vi "Evaluate.vi"(0 "object in":refnum<class "BallInterception.lvclass">, 2 "Point":dbl[](array[numeric]), 3 "Ally?":bool, 4 "GameRef":refnum<data-value>, 5 "error in (no error)":errorcluster) -> (14 "object out":refnum<class "BallInterception.lvclass">, 16 "Evaluation":dbl, 19 "error out":errorcluster)   [LabVIEW 2023, in "BallInterception.lvclass"]
uses:
  BallInterception.lvclass
  Game_class/Game.lvclass
  BallInterception.lvclass/BallInterception.ctl
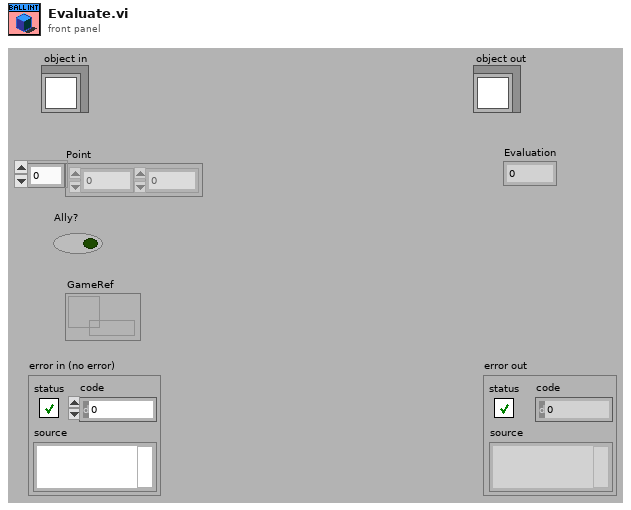
[diagram p1: front panel]
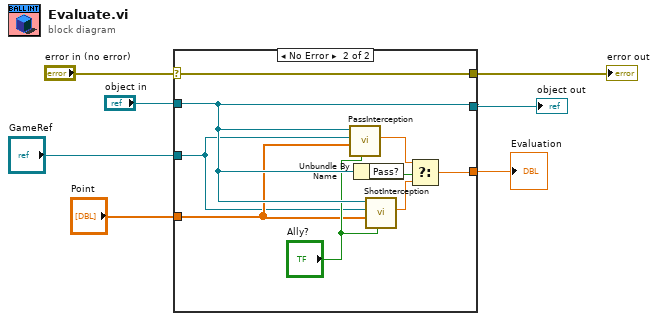
[diagram p0: block diagram]
diagram:
  n1 = case shown="No Error" "error in (no error)" {
    selector: "error in (no error)" -> [w9 w10]
    tunnel: [w9 w10] -> w6
    tunnel: "object in" -> [w8 w14]
    tunnel: [w8 w14] -> w4
    tunnel: "GameRef" -> [_ w11]
    tunnel: "Point" -> [_ w12]
    tunnel: [_ w15] -> w2
    frame Error {
    }
    frame No Error {
      n2 = call-dynamic "PassInterception.vi"("Ally?"="Ally?", "Point"=w12, "GameRef"=w11, "BallInterception in"=w14) -> ("Evaluation"=w16:dbl)  [unwired: 5 in, 2 out]
      n3 = Unbundle By Name(w14) -> ("Pass?"=w18:bool)
      n4 = call-dynamic "ShotInterception.vi"("Ally?"="Ally?", "Point"=w12, "GameRef"=w11, "BallInterception in"=w14) -> ("Evaluation"=w17:dbl)  [unwired: 5 in, 2 out]
      n5 = Select(t=w16, s=w18, f=w17) -> (s? t:f=w15:dbl)
    }
  }
  "error out" <- w6
  "object out" <- w4
  "Evaluation" <- w2
